vi "SFOAE-Compute Sweep Properties.vi"(0 "Sweep":T1, 5 "Level (dB SPL)":dbl, 7 "Cal File":path, 9 "Fs (Hz)":dbl, 11 "error in (no error)":errorcluster) -> (8 "sweep":dbl[](array[numeric]), 15 "error out":errorcluster)   [LabVIEW 2015]
uses:
  Typedefs/SFOAE-Sweep Params.ctl
  <vilib>/Analysis/4window.llb/windowTd.ctl
  Utility VIs/Math VIs/LinSpace (x0-dx-npts).vi
  <vilib>/Analysis/NI_AALPro.lvlib
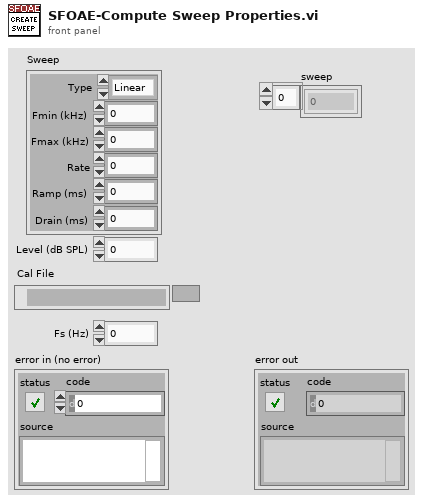
[diagram p1: front panel]
types:
  T1 = typedef "SFOAE-Sweep Params.ctl" = cluster{"Type":enum16{"Linear", "Log"}, "Fmin (kHz)":dbl, "Fmax (kHz)":dbl, "Rate":dbl, "Ramp (ms)":dbl, "Drain (ms)":dbl}
  T2 = typedef "NI_AALPro.lvlib/windowTd.ctl" = u32
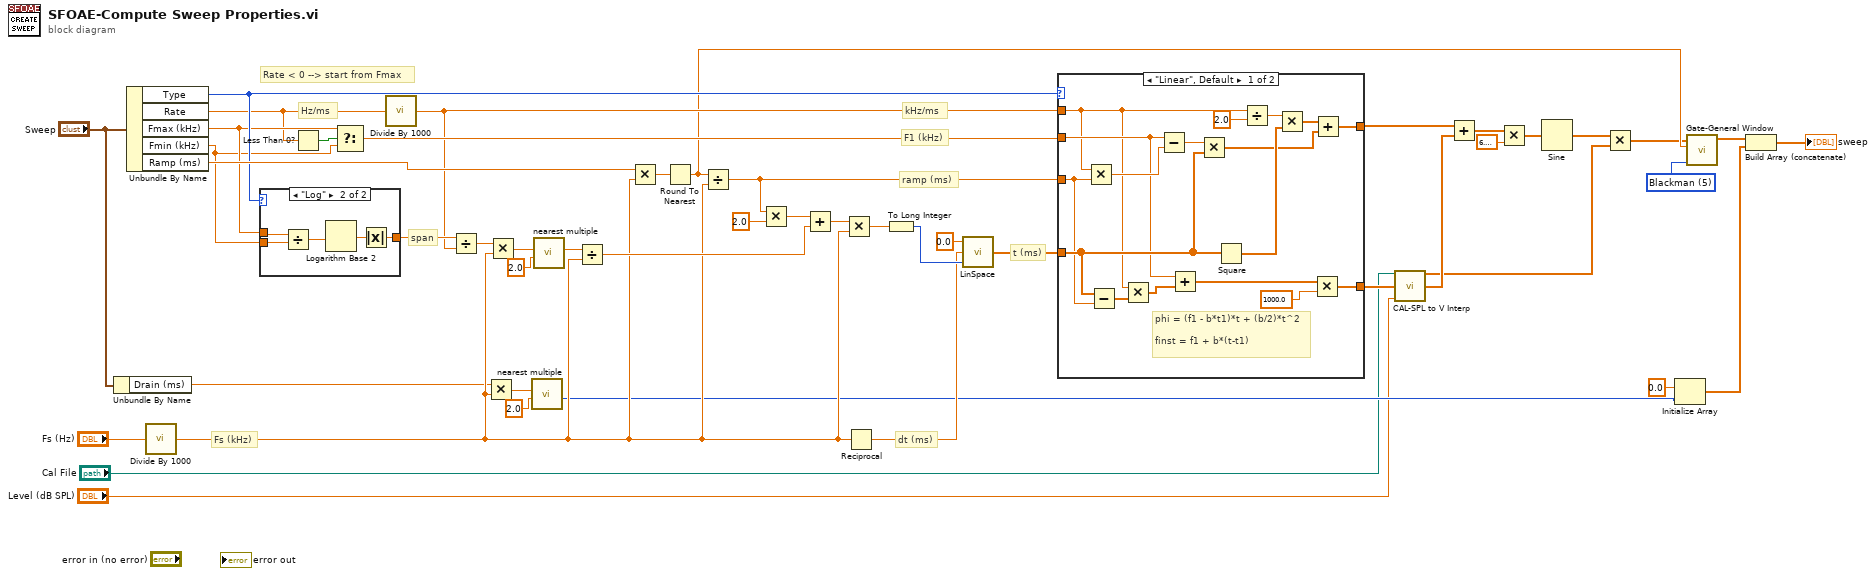
[diagram p0: block diagram]
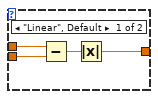
[diagram p3: hidden frame]
diagram:
  w19 = T2 5 items=["Rectangle"=0, "Hanning"=1, "Hamming"=2, "Blackman-Harris"=3, "Exact Blackman"=4, "Blackman"=5, "Flat Top"=6, "4 Term B-Harris "=7, "7 Term B-Harris"=8, "Low Sidelobe"=9, "Blackman Nuttall"=11, "Triangle"=30, "Bartlett-Hanning"=31, "Bohman"=32, "Parzen"=33, "Welch"=34, "Kaiser"=60, "Dolph-Chebyshev"=61, "Gaussian"=62] ("window")
  # "Hz/ms"
  # "Rate < 0 --> start from Fmax"
  # "F1 (kHz)"
  # "kHz/ms"
  # "ramp (ms)"
  # "t (ms)"
  # "dt (ms)"
  # "Fs (kHz)"
  # "span"
  n1 = Unbundle By Name("Sweep") -> ("Drain (ms)"=w12:dbl)
  n2 = Unbundle By Name("Sweep") -> ("Type"=w32:enum16{"Linear", "Log"}, "Rate"=w23:dbl, "Fmax (kHz)"=w29:dbl, "Fmin (kHz)"=w28:dbl, "Ramp (ms)"=w43:dbl)
  n3 = call "Divide By 1000.vi"("X"="Fs (Hz)") -> ("X/1000"=w14:dbl)
  n4 = case shown="\"Log\"" w32 {
    tunnel: w29 -> [w52 w56]
    tunnel: w28 -> [w51 w57]
    tunnel: [w49 w54] -> w48
    frame "Linear", Default {
      n5 = Subtract(x=w52, y=w51) -> (x-y=w50:dbl)
      n6 = Absolute Value(x=w50) -> (abs(x)=w49:dbl)
    }
    frame "Log" {
      n7 = Divide(x=w56, y=w57) -> (x/y=w55:dbl)
      n8 = Logarithm Base 2(1:w55) -> (0:w53:dbl)
      n9 = Absolute Value(x=w53) -> (abs(x)=w54:dbl)
    }
  }
  n10 = Less Than 0?(x=w23) -> (x < 0?=w30:bool)
  n11 = Select(t=w29, s=w30, f=w28) -> (s? t:f=w27:dbl)
  n12 = call "Divide By 1000.vi"("X"=w23) -> ("X/1000"=w22:dbl)
  n13 = Divide(x=w48, y=w22) -> (x/y=w47:dbl)
  n14 = Multiply(x=w12, y=w14) -> (x*y=w16:dbl)
  n15 = Multiply(x=w47, y=w14) -> (x*y=w46:dbl)
  n16 = call "nearest multiple.vi"("y"=2.0, "x"=w16) -> ("INT32(round(x/y)*y)"=w8:i32)  [unwired: 6 in, 1 out]
  n17 = call "nearest multiple.vi"("y"=2.0, "x"=w46) -> ("round(x/y)*y"=w44:dbl)  [unwired: 6 in, 1 out]
  n18 = Divide(x=w44, y=w14) -> (x/y=w39:dbl)
  n19 = Multiply(x=w43, y=w14) -> (x*y=w42:dbl)
  n20 = Round To Nearest(number=w42) -> (nearest integer value=w17:dbl)
  n21 = Divide(x=w17, y=w14) -> (x/y=w18:dbl)
  n22 = Multiply(x=w18, y=2.0) -> (x*y=w40:dbl)
  n23 = Add(x=w40, y=w39) -> (x+y=w38:dbl)
  n24 = Multiply(x=w38, y=w14) -> (x*y=w36:dbl)
  n25 = Reciprocal(x=w14) -> (1/x=w34:dbl)
  n26 = To Long Integer(number=w36) -> (32bit integer=w35:i32)
  n27 = call-poly "LinSpace.vi"("npts"=w35, "dx"=w34, "x0"=0.0) -> ("Array"=w31:dbl[])  [unwired: 1 in, 1 out]
  n28 = case shown="\"Linear\", Default" w32 {
    tunnel: w31 -> [w71 _]
    tunnel: w18 -> [w62 _]
    tunnel: w22 -> [w63 _]
    tunnel: w27 -> [w66 _]
    tunnel: [w59 _] -> w7
    tunnel: [w60 _] -> w26
    frame "Linear", Default {
      # "phi = (f1 - b*t1)*t + (b/2)*t^2\n\nfinst = f1 + b*(t-t1)"
      n29 = Multiply(x=w63, y=w62) -> (x*y=w74:dbl)
      n30 = Subtract(x=w71, y=w62) -> (x-y=w64:dbl[])
      n31 = Multiply(x=w63, y=w64) -> (x*y=w65:dbl[])
      n32 = Subtract(x=w66, y=w74) -> (x-y=w73:dbl)
      n33 = Add(x=w66, y=w65) -> (x+y=w61:dbl[])
      n34 = Multiply(x=w73, y=w71) -> (x*y=w67:dbl[])
      n35 = Square(x=w71) -> (x^2=w69:dbl[])
      n36 = Divide(x=w63, y=2.0) -> (x/y=w70:dbl)
      n37 = Multiply(x=w70, y=w69) -> (x*y=w68:dbl[])
      n38 = Multiply(x=w61, y=1000.0) -> (x*y=w59:dbl[])
      n39 = Add(x=w68, y=w67) -> (x+y=w60:dbl[])
    }
    frame "Log" {
    }
  }
  n40 = call "CAL-SPL to V Interp.vi"("user path"="Cal File", "Fi (Hz)"=w7, "dB SPL"="Level (dB SPL)") -> ("Amplitude (V)"=w2:dbl[], "Phase (cycles)"=w4:dbl[])  [unwired: 11 in]
  n41 = Add(x=w26, y=w4) -> (x+y=w5:dbl[])
  n42 = Multiply(x=w5, y=6.283185307179586) -> (x*y=w24:dbl[])
  n43 = Sine(x=w24) -> (sin(x)=w21:dbl[])
  n44 = Multiply(x=w21, y=w2) -> (x*y=w3:dbl[])
  n45 = Initialize Array(0.0 ("element"), w8) -> (w9:dbl[])
  n46 = call "Gate-General Window.vi"("window"=w19, "Nramp"=w17, "X"=w3) -> ("X windowed"=w20:dbl[])  [unwired: 8 in]
  n47 = Build Array (concatenate)(w20, w9) -> (→"sweep":dbl[])
